vi "Simulation Program.vi"() -> ()   [LabVIEW 2016]
panel:
  in  "Copy File Rate (s)":u32
  in  "Destination":path
  in  "Source Location":path
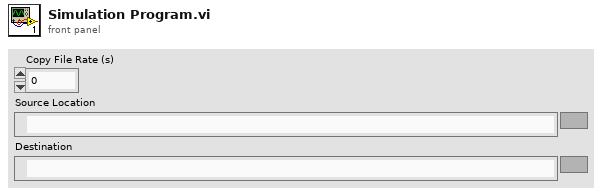
[diagram p1: front panel]
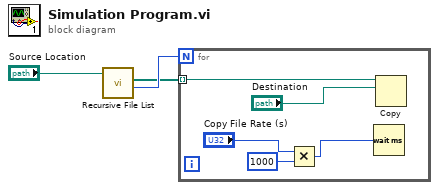
[diagram p0: block diagram]
diagram:
  n1 = call <vilib>:"Recursive File List.vi"("Folder Path"="Source Location") -> ("Number of Files"=w2:i32, "All Files in Dir"=w1:path[])  [unwired: 7 in, 2 out]
  n2 = for {
    N: w2 -> [_]
    tunnel: w1 -> [w8] mode=indexing
    n3 = Multiply(x="Copy File Rate (s)", y=u32 1000) -> (x*y=w5:u32)
    n4 = Wait (ms)(milliseconds to wait=w5) -> ()  [unwired: 1 out]
    n5 = Copy(10:"Destination", 11:w8) -> ()  [unwired: 3 in, 3 out]
  }
